vi "Read pmRA_masPYr.vi"(8 "error in (no error)":errorcluster, 11 "ProperMotion in":refnum<class "ProperMotion.lvclass">) -> (0 "error out":errorcluster, 2 "pmRA_masPYr":dbl[unit] min=-3.16878110868256e-07 max=3.16878110868256e-07, 3 "ProperMotion out":refnum<class "ProperMotion.lvclass">)   [LabVIEW 2014, in "TCSDataDefinitions.lvlib" / "TCSCommand.lvlib" / "TargetConfiguration.lvlib" / "Target.lvlib" / "FixedTarget.lvlib" / "ProperMotion.lvclass"]
uses:
  ProperMotion.lvclass
  ProperMotion.lvclass/ProperMotion.ctl
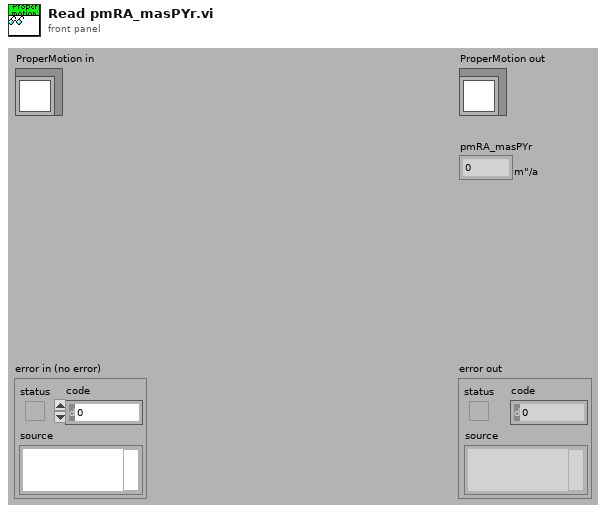
[diagram p1: front panel]
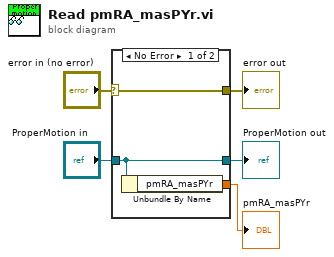
[diagram p0: block diagram]
diagram:
  n1 = case shown="No Error" "error in (no error)" {
    selector: "error in (no error)" -> [w8 w9]
    tunnel: [w8 w9] -> w4
    tunnel: [w7 w10] -> w2
    tunnel: "ProperMotion in" -> [w7 w10]
    tunnel: [w6 _] -> w1
    frame No Error {
      n2 = Unbundle By Name(w7) -> ("pmRA_masPYr"=w6:dbl[unit])
    }
    frame Error {
    }
  }
  "error out" <- w4
  "ProperMotion out" <- w2
  "pmRA_masPYr" <- w1
